vi "SbigQueryInfo.vi"(3 "Sbig":string, 9 "error in (no error)":errorcluster) -> (0 "Sbig out":string, 2 "Info":T1 {"Temperature Info"."Cooling %" format="%.2f"; "Temperature Info"."T Ambient" format="%.1f"; "Temperature Info"."T CCD" format="%.1f"; "Temperature Info"."T Setpoint" format="%.1f"}, 6 "error out":errorcluster)   [LabVIEW 2009]
uses:
  Controls/SbigStatus.ctl
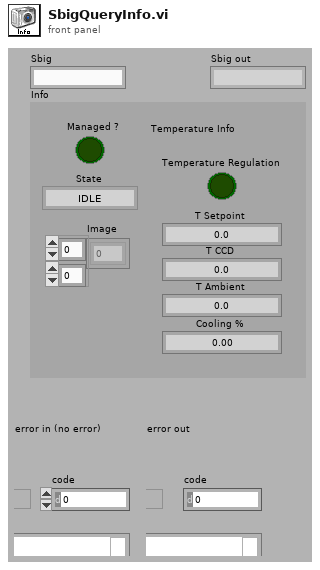
[diagram p1: front panel]
types:
  T1 = typedef "SbigStatus.ctl" = cluster{"Managed ?":bool, "State":enum16{"IDLE", "EXPOSING", "READING"}, "Image":i32[][], "Temperature Info":cluster{"Temperature Regulation":bool, "T Setpoint":dbl, "T CCD":dbl, "T Ambient":dbl, "Cooling %":dbl}}
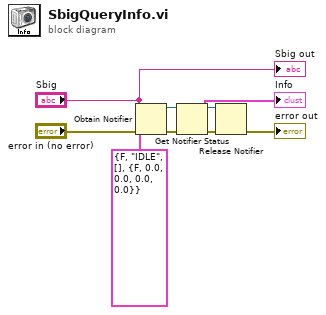
[diagram p0: block diagram]
diagram:
  n1 = Obtain Notifier(name (unnamed)="Sbig", notification data type=T1 {"Managed ?"=FALSE, "State"=enum."IDLE", "Image"=[], "Temperature Info"={"Temperature Regulation"=FALSE, "T Setpoint"=0.0, "T CCD"=0.0, "T Ambient"=0.0, "Cooling %"=0.0}} ("SbigStatus"), error in (no error)="error in (no error)") -> (notifier out=w5:refnum<notifier>, error out=w6:errorcluster)  [unwired: 1 in, 1 out]
  n2 = Get Notifier Status(notifier=w5, error in (no error)=w6) -> (notifier out=w8:refnum<notifier>, current notification=→"Info":T1, error out=w7:errorcluster)  [unwired: 2 out]
  n3 = Release Notifier(notifier=w8, error in (no error)=w7) -> (error out=→"error out":errorcluster)  [unwired: 3 out]
  "Sbig out" <- "Sbig"
